vi "Page_Web_Services_Initialize.vi"(6 "references":T1, 8 "error in (no error)":errorcluster, 11 "AB_Build in":refnum<class "AB_Build.lvclass">) -> (0 "error out":errorcluster, 3 "AB_Build out":refnum<class "AB_Build.lvclass">)   [LabVIEW 2020, in "AB_Build.lvclass"]
uses:
  <vilib>/AppBuilder/AB_Classes/Build/AB_Build.lvclass
  <resource>/Framework/Providers/Builds/AppBuilder/AB_UI_Page_Web_Services_References.ctl
  kernel32.dll
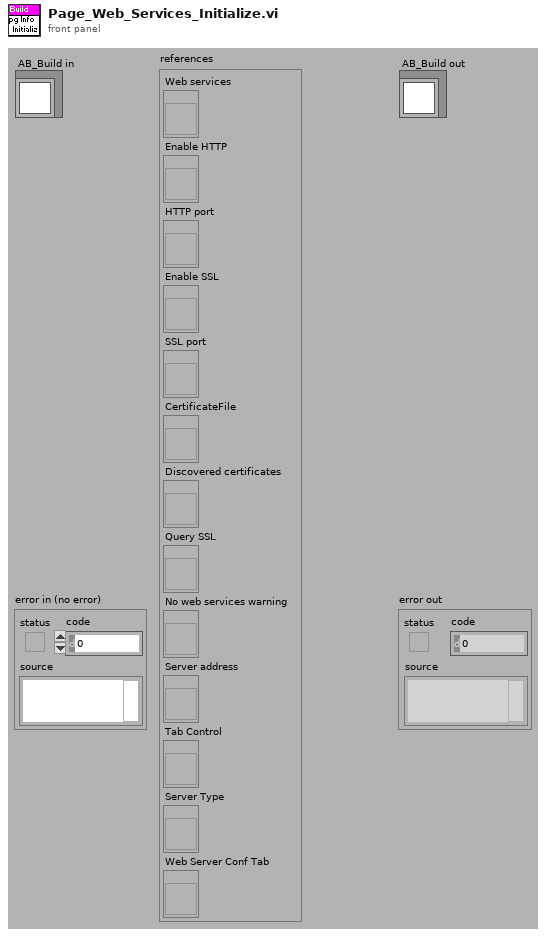
[diagram p1: front panel]
types:
  T1 = typedef "AB_UI_Page_Web_Services_References.ctl" = cluster{"Web services":refnum<vi>, "Enable HTTP":refnum<vi>, "HTTP port":refnum<vi>, "Enable SSL":refnum<vi>, "SSL port":refnum<vi>, "CertificateFile":refnum<vi>, "Discovered certificates":refnum<vi>, "Query SSL":refnum<vi>, "No web services warning":refnum<vi>, "Server address":refnum<vi>, "Tab Control":refnum<vi>, "Server Type":refnum<vi>, "Web Server Conf Tab":refnum<vi>}
  T2 = enum32{"NI Web Server", "Application Web Server"}
  T3 = typedef "LVRectTypeDef.ctl" = cluster{"Left":i16, "Top":i16, "Right":i16, "Bottom":i16}
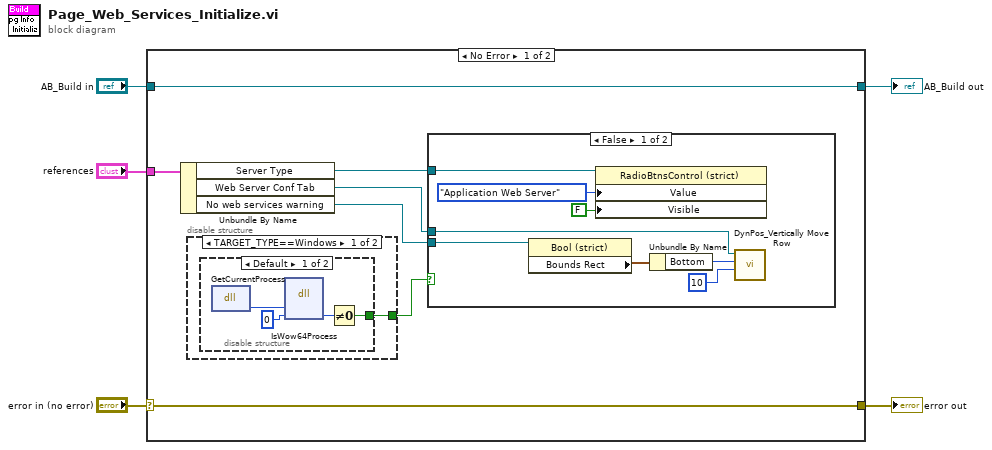
[diagram p0: block diagram]
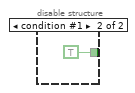
[diagram p2: hidden frame]
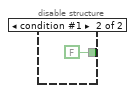
[diagram p3: hidden frame]
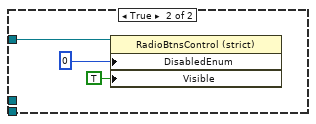
[diagram p4: hidden frame]
diagram:
  n1 = case shown="No Error" "error in (no error)" {
    selector: "error in (no error)" -> [w11 w32]
    tunnel: [w11 w32] -> w4
    tunnel: [w12 w31] -> w2
    tunnel: "AB_Build in" -> [w12 w31]
    tunnel: "references" -> [w9 _]
    frame No Error {
      n2 = Unbundle By Name(w9) -> ("Server Type"=w8:refnum<vi>, "Web Server Conf Tab"=w6:refnum<vi>, "No web services warning"=w7:refnum<vi>)
      n3 = disable-structure shown="TARGET_TYPE==Windows" {
        disable-tunnel: [w13 FALSE] -> w10
        frame condition #0 (active) {
          n4 = disable-structure shown="Default" {
            disable-tunnel: [w14 TRUE] -> w13
            frame condition #0 (active) {
              n5 = dll-call lib="kernel32.dll" fn="GetCurrentProcess"() -> ("return type"=w17:u64)  [unwired: 3 in, 2 out]
              n6 = dll-call lib="kernel32.dll" fn="IsWow64Process"("pid"=w17, "arg"=u32 0) -> ("arg"=w15:u32)  [unwired: 5 in, 2 out]
              n7 = Not Equal To 0?(x=w15) -> (x != 0?=w14:bool)
            }
            frame condition #1 {
            }
          }
        }
        frame condition #1 {
        }
      }
      n8 = case shown="False" w10 {
        tunnel: w8 -> [w26 w30]
        tunnel: w7 -> [w21 _]
        tunnel: w6 -> [w20 _]
        frame False {
          n9 = property class="Bool (strict)"(reference=w21) -> ("Bounds Rect"=w24:T3)  [unwired: 1 in, 2 out]
          n10 = property class="RadioBtnsControl (strict)"(reference=w26, "Value"=T2."Application Web Server", "Visible"=FALSE) -> ()  [unwired: 1 in, 2 out]
          n11 = Unbundle By Name(w24) -> ("Bottom"=w23:i16)
          n12 = call <vilib>:"DynPos_Vertically Move Row.vi"("Pixel separation (6)"=10, "Bottom of last control"=w23, "Control"=w20) -> ()  [unwired: 1 in, 8 out]
        }
        frame True {
          n13 = property class="RadioBtnsControl (strict)"(reference=w30, "DisabledEnum"=0, "Visible"=TRUE) -> ()  [unwired: 1 in, 2 out]
        }
      }
    }
    frame Error {
    }
  }
  "error out" <- w4
  "AB_Build out" <- w2
